vi "input.vi"(8 "error in":errorcluster, 10 "input allocation":T1, 11 "GPIC Core runtime in":refnum<class "GPIC Core runtime.lvclass">) -> (0 "error out":errorcluster, 2 "input data":T1, 3 "GPIC Core runtime out":refnum<class "GPIC Core runtime.lvclass">)   [LabVIEW 2017, in "GPIC Core runtime.lvclass"]
doc: "Provides an interface for reading data from a module at runtime. While this interface performs no operations, a child should provide an override which may read from any open sessions, references, or interfaces."
uses:
  GPIC Core runtime.lvclass
  <vilib>/NI/Tag Bus/table/data table.ctl
  GPIC Core runtime.lvclass/GPIC Core runtime.ctl
  CoreControlsRef.ctl
  <vilib>/NI/Tag Bus/table/data table.lvlib
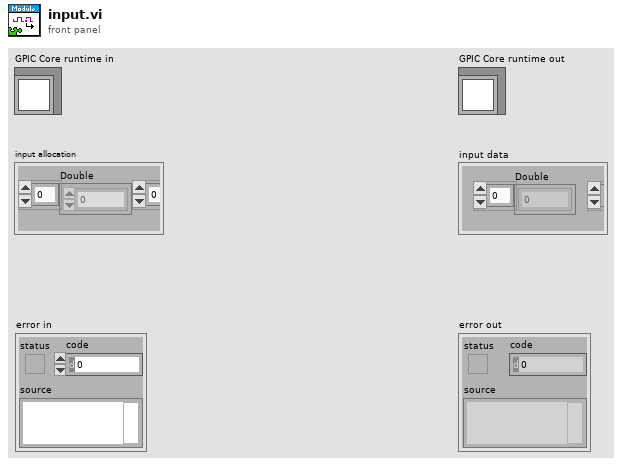
[diagram p1: front panel]
types:
  T1 = typedef "tag bus.lvlib/data table.lvlib/data table.ctl" = cluster{"Double":dbl[], "Single":sgl[], "I64":i64[], "I32":i32[], "I16":i16[], "I8":i8[], "U64":u64[], "U32":u32[], "U16":u16[], "U8":u8[], "Boolean":bool[], "String":string[], "Array of Double":cluster{"DBL Array":dbl[]}[], "Array of Single":cluster{"SGL Array":sgl[]}[], "Array of I64":cluster{"I64 Array":i64[]}[], "Array of I32":cluster{"I32 Array":i32[]}[], "Array of I16":cluster{"I16 Array":i16[]}[], "Array of I8":cluster{"I8 Array":i8[]}[], "Array of U64":cluster{"U64 Array":u64[]}[], "Array of U32":cluster{"U32 Array":u32[]}[], "Array of U16":cluster{"U16 Array":u16[]}[], "Array of U8":cluster{"U8 Array":u8[]}[], "Array of Boolean":cluster{"Boolean Array":bool[]}[], "Array of String":cluster{"String Array":string[]}[]}
  T2 = typedef "GPIC Core runtime.lvclass/CoreControlsRef.ctl" = refnum<k20>
  T3 = typedef "GPIC Core configuration.lvclass/input data indices.ctl" = cluster{"I16.AO_AO0":i32, "I16.AO_AO1":i32, "I16.AO_AO2":i32, "I16.AO_AO3":i32, "I16.AO_AO4":i32, "I16.AO_AO5":i32, "I16.AO_AO6":i32, "I16.AO_AO7":i32, "Boolean.HalfBridge_DO0":i32, "Boolean.HalfBridge_DO1":i32, "Boolean.HalfBridge_DO2":i32, "Boolean.HalfBridge_DO3":i32, "Boolean.HalfBridge_DO4":i32, "Boolean.HalfBridge_DO5":i32, "Boolean.HalfBridge_DO6":i32, "Boolean.HalfBridge_DO7":i32, "Boolean.HalfBridge_DO8":i32, "Boolean.HalfBridge_DO9":i32, "Boolean.HalfBridge_DO10":i32, "Boolean.HalfBridge_DO11":i32, "Boolean.HalfBridge_DO12":i32, "Boolean.HalfBridge_DO13":i32, "Boolean.LVTTL_DIO0":i32, "Boolean.LVTTL_DIO1":i32, "Boolean.LVTTL_DIO2":i32, "Boolean.LVTTL_DIO3":i32, "Boolean.LVTTL_DIO4":i32, "Boolean.LVTTL_DIO5":i32, "Boolean.LVTTL_DIO6":i32, "Boolean.LVTTL_DIO7":i32, "Boolean.LVTTL_DIO8":i32, "Boolean.LVTTL_DIO9":i32, "Boolean.LVTTL_DIO10":i32, "Boolean.LVTTL_DIO11":i32, "Boolean.LVTTL_DIO12":i32, "Boolean.LVTTL_DIO13":i32, "Boolean.LVTTL_DIO14":i32, "Boolean.LVTTL_DIO15":i32, "Boolean.LVTTL_DIO16":i32, "Boolean.LVTTL_DIO17":i32, "Boolean.LVTTL_DIO18":i32, "Boolean.LVTTL_DIO19":i32, "Boolean.LVTTL_DIO20":i32, "Boolean.LVTTL_DIO21":i32, "Boolean.LVTTL_DIO22":i32, "Boolean.LVTTL_DIO23":i32, "Boolean.LVTTL_DIO24":i32, "Boolean.LVTTL_DIO25":i32, "Boolean.LVTTL_DIO26":i32, "Boolean.LVTTL_DIO27":i32, "Boolean.LVTTL_DIO28":i32, "Boolean.LVTTL_DIO29":i32, "Boolean.LVTTL_DIO30":i32, "Boolean.LVTTL_DIO31":i32, "Boolean.RelayControl_DO0":i32, "Boolean.RelayControl_DO1":i32, "Boolean.RelayContro_DOl2":i32, "Boolean.RelayControl_DO3":i32, "Single.Scanned_AI0":i32, "Single.Scanned_AI1":i32, "Single.Scanned_AI2":i32, "Single.Scanned_AI3":i32, "Single.Scanned_AI4":i32, "Single.Scanned_AI5":i32, "Single.Scanned_AI6":i32, "Single.Scanned_AI7":i32, "Single.Simultaneous_AI0":i32, "Single.Simultaneous_AI1":i32, "Single.Simultaneous_AI2":i32, "Single.Simultaneous_AI3":i32, "Single.Simultaneous_AI4":i32, "Single.Simultaneous_AI5":i32, "Single.Simultaneous_AI6":i32, "Single.Simultaneous_AI7":i32, "Single.Simultaneous_AI8":i32, "Single.Simultaneous_AI9":i32, "Single.Simultaneous_AI10":i32, "Single.Simultaneous_AI11":i32, "Single.Simultaneous_AI12":i32, "Single.Simultaneous_AI13":i32, "Single.Simultaneous_AI14":i32, "Single.Simultaneous_AI15":i32, "Boolean.Sinking_DO0":i32, "Boolean.Sinking_DO1":i32, "Boolean.Sinking_DO2":i32, "Boolean.Sinking_DO3":i32, "Boolean.Sinking_DO4":i32, "Boolean.Sinking_DO5":i32, "Boolean.Sinking_DO6":i32, "Boolean.Sinking_DO7":i32, "Boolean.Sinking_DO8":i32, "Boolean.Sinking_DO9":i32, "Boolean.Sinking_DO10":i32, "Boolean.Sinking_DO11":i32, "Boolean.Sinking_DO12":i32, "Boolean.Sinking_DO13":i32, "Boolean.Sinking_DO14":i32, "Boolean.Sinking_DO15":i32, "Boolean.Sinking_DO16":i32, "Boolean.Sinking_DO17":i32, "Boolean.Sinking_DO18":i32, "Boolean.Sinking_DO19":i32, "Boolean.Sinking_DO20":i32, "Boolean.Sinking_DO21":i32, "Boolean.Sinking_DO22":i32, "Boolean.Sinking_DO23":i32, "Boolean.Sourcing_P0_DI0":i32, "Boolean.Sourcing_P0_DI1":i32, "Boolean.Sourcing_P0_DI2":i32, "Boolean.Sourcing_P0_DI3":i32, "Boolean.Sourcing_P0_DI4":i32, "Boolean.Sourcing_P0_DI5":i32, "Boolean.Sourcing_P0_DI6":i32, "Boolean.Sourcing_P0_DI7":i32, "Boolean.Sourcing_P0_DI8":i32, "Boolean.Sourcing_P0_DI9":i32, "Boolean.Sourcing_P0_DI10":i32, "Boolean.Sourcing_P0_DI11":i32, "Boolean.Sourcing_P0_DI12":i32, "Boolean.Sourcing_P0_DI13":i32, "Boolean.Sourcing_P1_DI0":i32, "Boolean.Sourcing_P1_DI1":i32, "Boolean.Sourcing_P1_DI2":i32, "Boolean.Sourcing_P1_DI3":i32, "Boolean.Sourcing_P1_DI4":i32, "Boolean.Sourcing_P1_DI5":i32, "Boolean.Sourcing_P1_DI6":i32, "Boolean.Sourcing_P1_DI7":i32, "Boolean.Sourcing_P1_DI8":i32, "Boolean.Sourcing_P1_DI9":i32, "Boolean.Sourcing_P1_DI10":i32, "Boolean.Sourcing_P1_DI11":i32, "Boolean.Sourcing_P1_DI12":i32, "Boolean.Sourcing_P1_DI13":i32}
  T4 = typedef "GPIC Core runtime.lvclass/input user data.ctl" = cluster{"AO_AO0":i16, "AO_AO1":i16, "AO_AO2":i16, "AO_AO3":i16, "AO_AO4":i16, "AO_AO5":i16, "AO_AO6":i16, "AO_AO7":i16, "HalfBridge_DO0":bool, "HalfBridge_DO1":bool, "HalfBridge_DO2":bool, "HalfBridge_DO3":bool, "HalfBridge_DO4":bool, "HalfBridge_DO5":bool, "HalfBridge_DO6":bool, "HalfBridge_DO7":bool, "HalfBridge_DO8":bool, "HalfBridge_DO9":bool, "HalfBridge_DO10":bool, "HalfBridge_DO11":bool, "HalfBridge_DO12":bool, "HalfBridge_DO13":bool, "LVTTL_DIO0":bool, "LVTTL_DIO1":bool, "LVTTL_DIO2":bool, "LVTTL_DIO3":bool, "LVTTL_DIO4":bool, "LVTTL_DIO5":bool, "LVTTL_DIO6":bool, "LVTTL_DIO7":bool, "LVTTL_DIO8":bool, "LVTTL_DIO9":bool, "LVTTL_DIO10":bool, "LVTTL_DIO11":bool, "LVTTL_DIO12":bool, "LVTTL_DIO13":bool, "LVTTL_DIO14":bool, "LVTTL_DIO15":bool, "LVTTL_DIO16":bool, "LVTTL_DIO17":bool, "LVTTL_DIO18":bool, "LVTTL_DIO19":bool, "LVTTL_DIO20":bool, "LVTTL_DIO21":bool, "LVTTL_DIO22":bool, "LVTTL_DIO23":bool, "LVTTL_DIO24":bool, "LVTTL_DIO25":bool, "LVTTL_DIO26":bool, "LVTTL_DIO27":bool, "LVTTL_DIO28":bool, "LVTTL_DIO29":bool, "LVTTL_DIO30":bool, "LVTTL_DIO31":bool, "RelayControl_DO0":bool, "RelayControl_DO1":bool, "RelayContro_DOl2":bool, "RelayControl_DO3":bool, "Scanned_AI0":sgl, "Scanned_AI1":sgl, "Scanned_AI2":sgl, "Scanned_AI3":sgl, "Scanned_AI4":sgl, "Scanned_AI5":sgl, "Scanned_AI6":sgl, "Scanned_AI7":sgl, "Simultaneous_AI0":sgl, "Simultaneous_AI1":sgl, "Simultaneous_AI2":sgl, "Simultaneous_AI3":sgl, "Simultaneous_AI4":sgl, "Simultaneous_AI5":sgl, "Simultaneous_AI6":sgl, "Simultaneous_AI7":sgl, "Simultaneous_AI8":sgl, "Simultaneous_AI9":sgl, "Simultaneous_AI10":sgl, "Simultaneous_AI11":sgl, "Simultaneous_AI12":sgl, "Simultaneous_AI13":sgl, "Simultaneous_AI14":sgl, "Simultaneous_AI15":sgl, "Sinking_DO0":bool, "Sinking_DO1":bool, "Sinking_DO2":bool, "Sinking_DO3":bool, "Sinking_DO4":bool, "Sinking_DO5":bool, "Sinking_DO6":bool, "Sinking_DO7":bool, "Sinking_DO8":bool, "Sinking_DO9":bool, "Sinking_DO10":bool, "Sinking_DO11":bool, "Sinking_DO12":bool, "Sinking_DO13":bool, "Sinking_DO14":bool, "Sinking_DO15":bool, "Sinking_DO16":bool, "Sinking_DO17":bool, "Sinking_DO18":bool, "Sinking_DO19":bool, "Sinking_DO20":bool, "Sinking_DO21":bool, "Sinking_DO22":bool, "Sinking_DO23":bool, "Sourcing_P0_DI0":bool, "Sourcing_P0_DI1":bool, "Sourcing_P0_DI2":bool, "Sourcing_P0_DI3":bool, "Sourcing_P0_DI4":bool, "Sourcing_P0_DI5":bool, "Sourcing_P0_DI6":bool, "Sourcing_P0_DI7":bool, "Sourcing_P0_DI8":bool, "Sourcing_P0_DI9":bool, "Sourcing_P0_DI10":bool, "Sourcing_P0_DI11":bool, "Sourcing_P0_DI12":bool, "Sourcing_P0_DI13":bool, "Sourcing_P1_DI0":bool, "Sourcing_P1_DI1":bool, "Sourcing_P1_DI2":bool, "Sourcing_P1_DI3":bool, "Sourcing_P1_DI4":bool, "Sourcing_P1_DI5":bool, "Sourcing_P1_DI6":bool, "Sourcing_P1_DI7":bool, "Sourcing_P1_DI8":bool, "Sourcing_P1_DI9":bool, "Sourcing_P1_DI10":bool, "Sourcing_P1_DI11":bool, "Sourcing_P1_DI12":bool, "Sourcing_P1_DI13":bool}
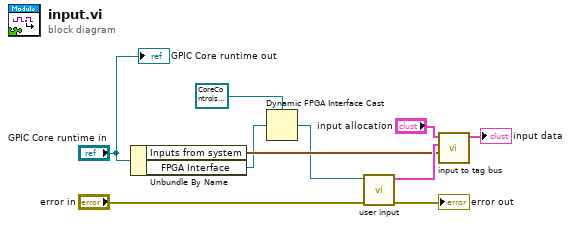
[diagram p0: block diagram]
diagram:
  n1 = Unbundle By Name("GPIC Core runtime in") -> ("Inputs from system"=w5:T3, "FPGA Interface"=w4:refnum<k20>)
  n2 = Dynamic FPGA Interface Cast(Session In=T2 refnum ("FPGA Interface"), Type=w4) -> (Session Out=w2:T2)
  n3 = call "user input.vi"("error in"="error in", "FPGA Interface"=w2) -> ("error out"=→"error out":errorcluster, "Inputs from system"=w6:T4)  [unwired: 8 in]
  n4 = call "input to tag bus.vi"("indices"=w5, "data cluster"=w6, "tag bus in"="input allocation") -> ("tag bus out"=→"input data":T1)  [unwired: 8 in]
  "GPIC Core runtime out" <- "GPIC Core runtime in"
